vi "Ctrls state & value on Start-Stop.vi"(8 "error in (no error)":errorcluster, 11 "Queue data":T1) -> (0 "error out":errorcluster)   [LabVIEW 2017]
uses:
  Typedefs/Next state queue data.ctl
  Typedefs/Start-Stop Enum.ctl
  Typedefs/Top level VI states.ctl
  Typedefs/Read Write Enum.ctl
  Typedefs/Set Main VI cursor.ctl
  Global Variables/gl_UI Ctrl Refs.vi
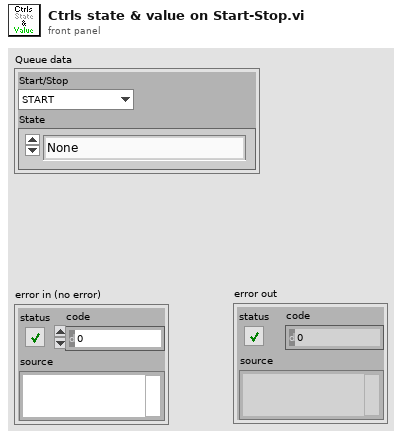
[diagram p1: front panel]
types:
  T1 = typedef "Next state queue data.ctl" = cluster{"Start/Stop":T2, "State":T3}
  T2 = typedef "Start-Stop Enum.ctl" = enum16{"START", "STOP"}
  T3 = typedef "Top level VI states.ctl" = enum16{"None", "Initialise UI", "<STACK PROTOCOL STATES>", "AOL Zstack-START", "AOL Zstack-STOP", "Motor Zstack-START", "Motor Zstack-STOP", "<ACQUISITION PROTOCOL STATES> ", "Functional Acquisition-START", "Functional Acquisition-STOP", "Single Plane Acquisition-START", "Single Plane Acquisition-STOP", "Volume Acquisition-START", "Volume Acquisition-STOP", "<LIVE IMAGING PROTOCOL STATES>", "Live Imaging-START", "Live Imaging-STOP", "Live Plane Imaging-START", "Live Plane Imaging-STOP", "Live Volume Imaging-START", "Live Volume Imaging-STOP", "<MOVEMENT CORRECTION PROTOCOL STATES>", "EXIT"}
  T4 = enum8{"Enabled", "Disabled", "Disabled and Grayed Out"}
  T5 = typedef "Read Write Enum.ctl" = enum16{"Read", "Write"}
  T6 = typedef "UI ctrl refs cluster.ctl" = cluster{"Top level VI path":path, "Top level VI ref":refnum<vi>, "User menu ref":refnum<k9>, "Sub Panel control":refnum<vi>, "Imaging Param Tab":refnum<vi>, "Occurrence-Start drivers":refnum<k4>, "Occurrence-Speed logging initialised":refnum<k4>, "Occurrence-XYZ stage initialised":refnum<k4>, "Exit button":refnum<vi>, "Status ind":refnum<vi>, "Set as origin":refnum<vi>, "Speed Logging":refnum<vi>, "Time Lapse":refnum<vi>, "Live Imaging":refnum<vi>, "AOL Z Stack":refnum<vi>, "Motor Z Stack":refnum<vi>, "Funct Acq button":refnum<vi>, "Hard Shutter":refnum<vi>, "Virtual Shutter":refnum<vi>, "Laser Power":refnum<vi>, "AOL Mode":refnum<vi>, "Frame Size":refnum<vi>, "Field of View":refnum<vi>, "Dwell Time":refnum<vi>, "Zoom":refnum<vi>, "AOL Z":refnum<vi>, "Objective":refnum<vi>, "Axis":refnum<vi>, "Paths & Names":refnum<vi>, "Experiment folder path (ind.)":refnum<vi>, "Last State (Ind.)":refnum<vi>, "Averages":refnum<vi>, "Angle (degrees)":refnum<vi>, "X centre":refnum<vi>, "Y centre":refnum<vi>, "Plane Mode":refnum<vi>, "# Planes":refnum<vi>, "Z Start":refnum<vi>, "Z Stop":refnum<vi>, "Z Step":refnum<vi>, "PMT 1":refnum<vi>, "PMT 2":refnum<vi>, "Stage XYZ Position":refnum<vi>, "Pockels@Z Start":refnum<vi>, "Pockels@Z Stop":refnum<vi>, "Obtain Z Start":refnum<vi>, "Obtain Z Stop":refnum<vi>, "Live stim.trig.period":refnum<vi>, "Live stim.trig.enable":refnum<vi>, "XY Stage Move":refnum<vi>, "Funct. Acq. Pockels Modulation":refnum<vi>, "Enable Video Recording":refnum<vi>, "Video Record-Live Imaging":refnum<vi>, "Video Record-Funct acq":refnum<vi>, "AOL Z-stack Chirps Ready (ind)":refnum<vi>, "Target time between mov.cor. ref triggers (ms)":refnum<vi>, "Funct. Acq. Ref frame save":refnum<vi>, "Show ref plots window":refnum<vi>, "Center freq ind (nm)":refnum<vi>, "Pickup mode (ind)":refnum<vi>, "Logging queue (ind)":refnum<vi>, "Back aperture power (ind.)":refnum<vi>, "Power after objective (ind.)":refnum<vi>, "Switch user":refnum<vi>, "Ls1 Conn. Status":refnum<vi>, "Ls1Tuning Status":refnum<vi>, "Ls1 Faults":refnum<vi>, "Ls1 Connection":refnum<vi>, "Ls1 Mode":refnum<vi>, "Ls1 POWER [mW]":refnum<vi>, "Ls1Shutter":refnum<vi>, "Ls1 Wavelength":refnum<vi>, "Ls1 Note":refnum<vi>, "Ls1 Confirm Wav":refnum<vi>, "Ls1 PreChrp Prism1":refnum<vi>, "Ls1 PreChrp Prism2":refnum<vi>, "Ls1 wav top Ind":refnum<vi>, "Ls1 power top Ind":refnum<vi>, "Ls1 Pump peak Hold":refnum<vi>, "Ls1 Status Ind":refnum<vi>, "Ls1 wav cancel":refnum<vi>, "Experiment Type":refnum<vi>, "Biology Information":refnum<vi>}
  T7 = typedef "Set Main VI cursor.ctl" = enum16{"Release busy cursor", "Set busy cursor"}
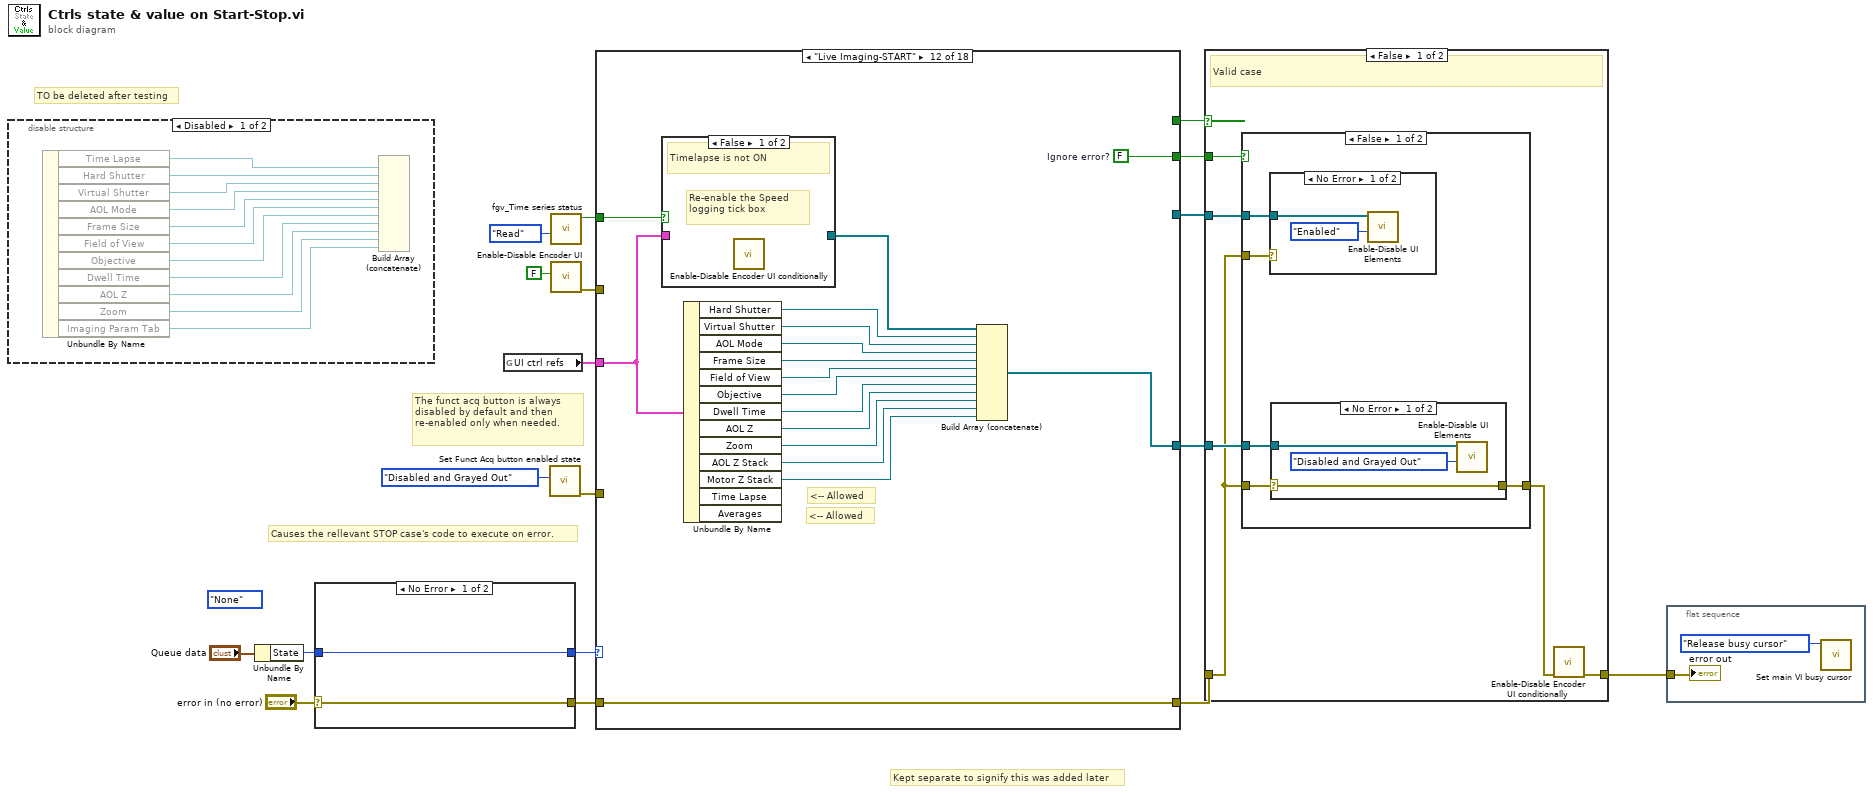
[diagram p0: block diagram]
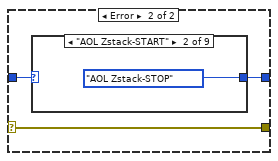
[diagram p3: hidden frame]
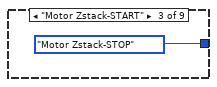
[diagram p5: hidden frame]
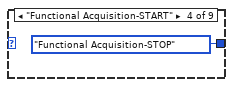
[diagram p6: hidden frame]
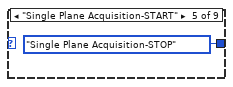
[diagram p7: hidden frame]
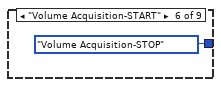
[diagram p8: hidden frame]
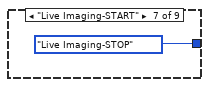
[diagram p9: hidden frame]
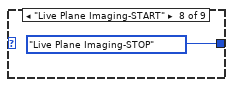
[diagram p10: hidden frame]
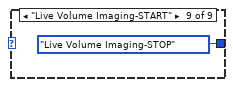
[diagram p11: hidden frame]
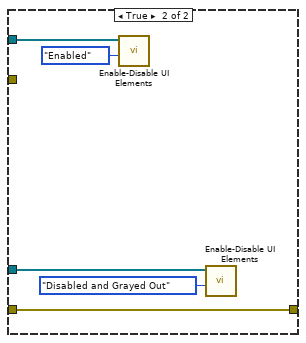
[diagram p14: hidden frame]
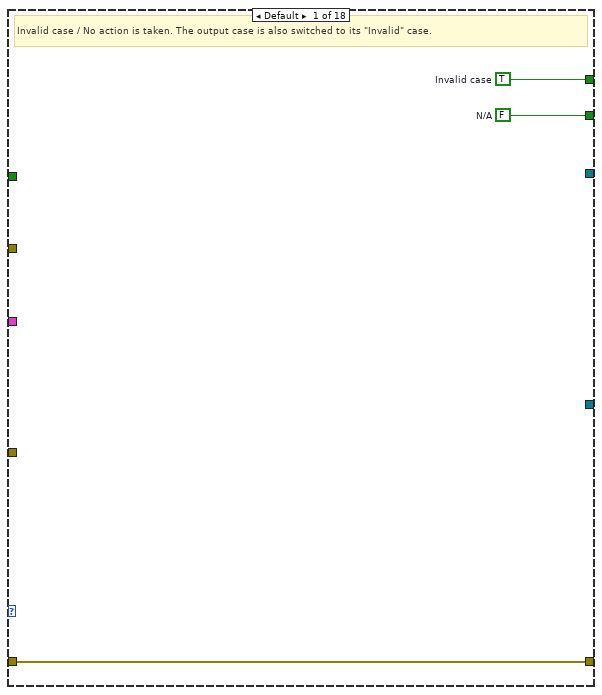
[diagram p16: hidden frame]
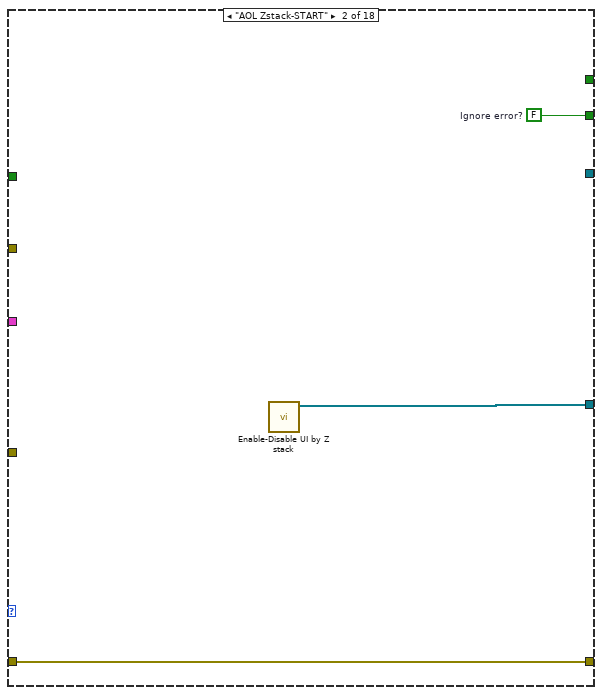
[diagram p17: hidden frame]
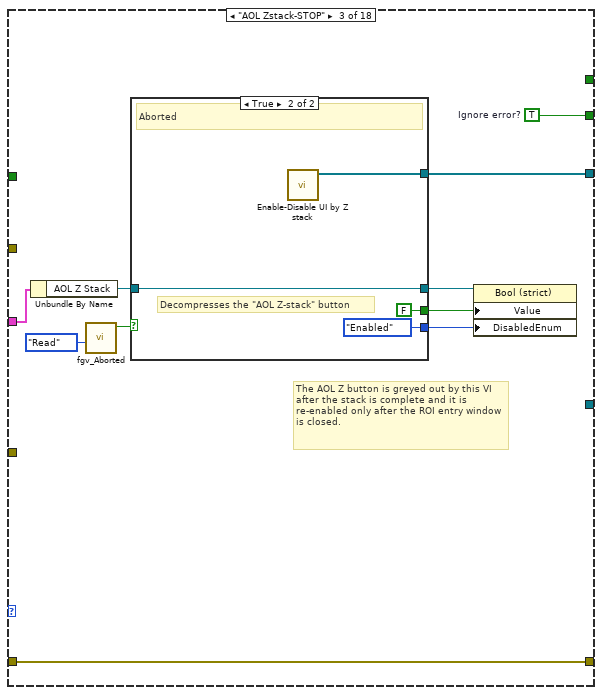
[diagram p18: hidden frame]
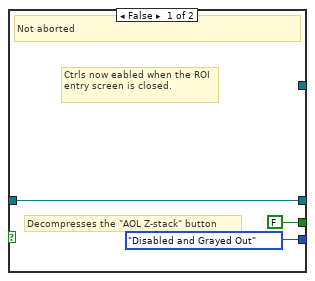
[diagram p19: hidden frame]
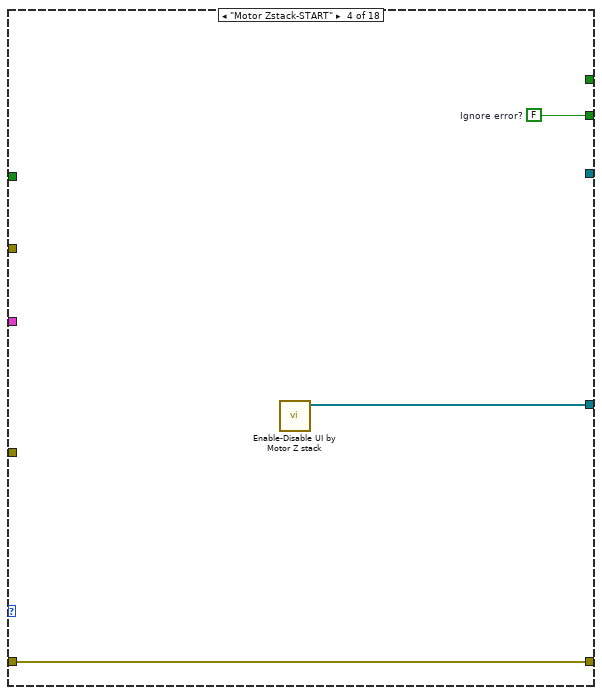
[diagram p20: hidden frame]
diagram:
  (unwired) Top_level_VI_states."None" ("State")
  # "TO be deleted after testing"
  # "Kept separate to signify this was added later"
  # "The funct acq button is always disabled by default and then re-enabled only when needed."
  # "Causes the rellevant STOP case's code to execute on error."
  n1 = disable-structure shown="Disabled" {
    frame Disabled {
      n2 = Unbundle By Name() -> ("Time Lapse"=w20:refnum<vi>, "Hard Shutter"=w22:refnum<vi>, "Virtual Shutter"=w23:refnum<vi>, "AOL Mode"=w24:refnum<vi>, "Frame Size"=w25:refnum<vi>, "Field of View"=w26:refnum<vi>, "Objective"=w27:refnum<vi>, "Dwell Time"=w28:refnum<vi>, "AOL Z"=w29:refnum<vi>, "Zoom"=w30:refnum<vi>, "Imaging Param Tab"=w21:refnum<vi>)  [unwired: 1 in]
      n3 = Build Array (concatenate)(w20, w22, w23, w24, w25, w26, w27, w28, w29, w30, w21) -> (w19:refnum<vi>[])  [unwired: 1 out]
    }
    frame Enabled {
    }
  }
  n4 = Unbundle By Name("Queue data") -> ("State"=w10:T3)
  n5 = case shown="No Error" "error in (no error)" {
    selector: "error in (no error)" -> [w31 w35]
    tunnel: w10 -> [w32 w34]
    tunnel: [w32 w33] -> w8
    tunnel: [w31 w35] -> w4
    frame No Error {
    }
    frame Error {
      n6 = case shown="\"AOL Zstack-START\"" w34 {
        selector: w34 -> [w36 _ _ _ _ _ _ _ _]
        tunnel: [w36 Top_level_VI_states."AOL Zstack-STOP" ("State") Top_level_VI_states."Motor Zstack-STOP" ("State") Top_level_VI_states."Functional Acquisition-STOP" ("State") Top_level_VI_states."Single Plane Acquisition-STOP" ("State") Top_level_VI_states."Volume Acquisition-STOP" ("State") Top_level_VI_states."Live Imaging-STOP" ("State") Top_level_VI_states."Live Plane Imaging-STOP" ("State") Top_level_VI_states."Live Volume Imaging-STOP" ("State")] -> w33
        frame Default {
        }
        frame "AOL Zstack-START" {
        }
        frame "Motor Zstack-START" {
        }
        frame "Functional Acquisition-START" {
        }
        frame "Single Plane Acquisition-START" {
        }
        frame "Volume Acquisition-START" {
        }
        frame "Live Imaging-START" {
        }
        frame "Live Plane Imaging-START" {
        }
        frame "Live Volume Imaging-START" {
        }
      }
    }
  }
  n7 = global read "gl_UI Ctrl Refs.vi" "UI ctrl refs"() -> (w18:T6)
  n8 = call "Set Funct Acq button enabled state.vi"("Disabled"=T4."Disabled and Grayed Out") -> ("error out"=w6:errorcluster)  [unwired: 10 in]
  n9 = call "fgv_Time series status.vi"("Function"=Read_Write_Enum."Read") -> ("Timelapse?"=w11:bool)  [unwired: 10 in]
  n10 = call "Enable-Disable Encoder UI.vi"("Cam VidRec.VidRec available"=FALSE) -> ("error out"=w1:errorcluster)  [unwired: 10 in]
  n11 = case "Message Cases" shown="\"Live Imaging-START\"" w8 {
    tunnel: w18 -> [_ _ w53 _ w72 w91 w112 w132 w151 w170 w188 w205 w224 w242 w259 w273 w291 w306]
    tunnel: [_ _ w56 _ w71 _ w122 _ w160 _ w186 _ w232 _ w263 _ w294 _] -> w17
    tunnel: [w47 _ _ _ _ _ _ _ _ _ _ _ _ _ _ _ _ _] -> w15
    tunnel: [_ w49 _ w70 _ w93 _ w141 _ w176 _ w213 _ w247 _ w278 _ w308] -> w14
    tunnel: [w46 w50 w60 w69 w80 w92 w121 w140 w159 w175 w204 w212 w231 w246 w262 w277 w293 w307] -> w13
    tunnel: w11 -> [_ _ _ _ _ _ _ _ _ _ _ w208 _ w245 _ w276 _ w305]
    tunnel: w6 -> [_ _ _ _ _ _ _ _ _ _ _ _ _ _ _ _ _ _]
    tunnel: w4 -> [w45 w48 w59 w68 w79 w88 w113 w133 w152 w171 w203 w206 w225 w243 w260 w274 w292 w304]
    tunnel: [w45 w48 w59 w68 w79 w88 w113 w133 w152 w171 w203 w206 w225 w243 w260 w274 w292 w304] -> w3
    tunnel: w1 -> [_ _ _ _ _ _ _ _ _ _ _ _ _ _ _ _ _ _]
    frame Default {
      w46 = FALSE  # N/A
      w47 = TRUE  # Invalid case
      # "Invalid case / No action is taken. The output case is also switched to its \"Invalid\" case."
    }
    frame "AOL Zstack-START" {
      w50 = FALSE  # Ignore error?
      n12 = call "Enable-Disable UI by Z stack.vi"() -> ("Controls refs to enable/disable"=w49:refnum<vi>[])  [unwired: 11 in]
    }
    frame "AOL Zstack-STOP" {
      w60 = TRUE  # Ignore error?
      # "The AOL Z button is greyed out by this VI after the stack is complete and it is re-enabled only after the ROI entry window is closed."
      n13 = Unbundle By Name(w53) -> ("AOL Z Stack"=w52:refnum<vi>)
      n14 = call "fgv_Aborted.vi"("Function"=Read_Write_Enum."Read") -> ("Funct Acq Aborted?"=w57:bool)  [unwired: 9 in, 1 out]
      n15 = case shown="True" w57 {
        tunnel: [_ w67] -> w56
        tunnel: [FALSE ("Value") FALSE ("Value")] -> w55
        tunnel: [T4."Disabled and Grayed Out" ("Disabled") T4."Enabled" ("Disabled")] -> w54
        tunnel: w52 -> [w62 w66]
        tunnel: [w62 w66] -> w51
        frame False {
          # "Ctrls now eabled when the ROI entry screen is closed."
          # "Decompresses the \"AOL Z-stack\" button"
          # "Not aborted"
        }
        frame True {
          # "Decompresses the \"AOL Z-stack\" button"
          # "Aborted"
          n16 = call "Enable-Disable UI by Z stack.vi"() -> ("Controls refs to enable/disable"=w67:refnum<vi>[])  [unwired: 11 in]
        }
      }
      n17 = property class="Bool (strict)"(reference=w51, "Value"=w55, "DisabledEnum"=w54) -> ()  [unwired: 1 in, 2 out]
    }
    frame "Motor Zstack-START" {
      w69 = FALSE  # Ignore error?
      n18 = call "Enable-Disable UI by Motor Z stack.vi"() -> ("Controls to disable"=w70:refnum<vi>[])  [unwired: 11 in]
    }
    frame "Motor Zstack-STOP" {
      w80 = TRUE  # Ignore error?
      # "The Motor Z button is greyed out by this VI after the stack is complete and it is re-enabled only after the ROI entry window is closed."
      n19 = Unbundle By Name(w72) -> ("Motor Z Stack"=w77:refnum<vi>)
      n20 = call "fgv_Aborted.vi"("Function"=Read_Write_Enum."Read") -> ("Funct Acq Aborted?"=w74:bool)  [unwired: 9 in, 1 out]
      n21 = case shown="False" w74 {
        tunnel: [_ w84] -> w71
        tunnel: [FALSE ("Value") FALSE ("Value")] -> w75
        tunnel: [T4."Disabled and Grayed Out" ("Disabled") T4."Enabled" ("Disabled")] -> w76
        tunnel: w77 -> [w82 w87]
        tunnel: [w82 w87] -> w78
        frame False {
          # "Ctrls now eabled when the ROI entry screen is closed."
          # "Decompresses the \"AOL Z-stack\" button"
          # "Not aborted"
        }
        frame True {
          # "Decompresses the \"Motor Z-stack\" button"
          # "Aborted"
          n22 = call "Enable-Disable UI by Motor Z stack.vi"() -> ("Controls to disable"=w84:refnum<vi>[])  [unwired: 11 in]
        }
      }
      n23 = property class="Bool (strict)"(reference=w78, "Value"=w75, "DisabledEnum"=w76) -> ()  [unwired: 1 in, 2 out]
    }
    frame "Functional Acquisition-START" {
      w92 = FALSE  # Ignore error?
      # "The funct acq button's state is explicitly set by this VI, throughout the software."
      n24 = call "Set Funct Acq button enabled state.vi"("Disabled"=T4."Enabled") -> ("error out"=w89:errorcluster)  [unwired: 10 in]
      n25 = flat-sequence {
        tunnel: [w110] -> w93
        tunnel: w91 -> [w94]
        tunnel: w89 -> [_]
        frame #0 {
          n26 = Unbundle By Name(w94) -> ("Time Lapse"=w99:refnum<vi>, "Imaging Param Tab"=w100:refnum<vi>, "Hard Shutter"=w101:refnum<vi>, "Virtual Shutter"=w102:refnum<vi>, "AOL Mode"=w103:refnum<vi>, "Frame Size"=w104:refnum<vi>, "Field of View"=w105:refnum<vi>, "Objective"=w106:refnum<vi>, "Dwell Time"=w107:refnum<vi>, "AOL Z"=w108:refnum<vi>, "Zoom"=w109:refnum<vi>, "Live Imaging"=w97:refnum<vi>, "AOL Z Stack"=w96:refnum<vi>, "Motor Z Stack"=w95:refnum<vi>)
          n27 = call "Time series conditional disable ctrl refs.vi"("UI ctrl refs"=w94) -> ("Ctrl refs"=w98:refnum<vi>[])  [unwired: 10 in]
          n28 = Build Array (concatenate)(w98, w99, w100, w101, w102, w103, w104, w105, w106, w107, w108, w109, w97, w96, w95) -> (w110:refnum<vi>[])
        }
      }
    }
    frame "Functional Acquisition-STOP" {
      w121 = TRUE  # Ignore error?
      # "Decompresses the \"funct. acq.\" button"
      # "Controls enabled when Live Imaging is stopped"
      n29 = Unbundle By Name(w112) -> ("Time Lapse"=w119:refnum<vi>, "Hard Shutter"=w123:refnum<vi>, "Virtual Shutter"=w124:refnum<vi>, "AOL Mode"=w125:refnum<vi>, "Frame Size"=w126:refnum<vi>, "Field of View"=w127:refnum<vi>, "Objective"=w128:refnum<vi>, "Dwell Time"=w129:refnum<vi>, "AOL Z"=w130:refnum<vi>, "Zoom"=w131:refnum<vi>, "Imaging Param Tab"=w120:refnum<vi>, "Live Imaging"=w118:refnum<vi>, "AOL Z Stack"=w117:refnum<vi>, "Motor Z Stack"=w116:refnum<vi>)
      n30 = call "Time series conditional disable ctrl refs.vi"("UI ctrl refs"=w112) -> ("Ctrl refs"=w111:refnum<vi>[])  [unwired: 10 in]
      n31 = call "Set Funct Acq button value.vi"("Functional Acquisition button's new value"=FALSE ("Value")) -> ()  [unwired: 10 in, 1 out]
      n32 = call "Set Funct Acq button enabled state.vi"("Disabled"=T4."Enabled") -> ()  [unwired: 10 in, 1 out]
      n33 = Build Array (concatenate)(w119, w123, w124, w125, w126, w127, w128, w129, w130, w131, w120, w118, w117, w116, w111) -> (w122:refnum<vi>[])
    }
    frame "Single Plane Acquisition-START" {
      w140 = FALSE  # Ignore error?
      # "Not in use - placeholder only"
      n34 = Unbundle By Name(w132) -> ("Time Lapse"=w138:refnum<vi>, "Imaging Param Tab"=w139:refnum<vi>, "Hard Shutter"=w142:refnum<vi>, "Virtual Shutter"=w143:refnum<vi>, "AOL Mode"=w144:refnum<vi>, "Frame Size"=w145:refnum<vi>, "Field of View"=w146:refnum<vi>, "Objective"=w147:refnum<vi>, "Dwell Time"=w148:refnum<vi>, "AOL Z"=w149:refnum<vi>, "Zoom"=w150:refnum<vi>, "AOL Z Stack"=w136:refnum<vi>, "Motor Z Stack"=w135:refnum<vi>, "Live Imaging"=w134:refnum<vi>)
      n35 = call "Time series conditional disable ctrl refs.vi"("UI ctrl refs"=w132) -> ("Ctrl refs"=w137:refnum<vi>[])  [unwired: 10 in]
      n36 = Build Array (concatenate)(w137, w138, w139, w142, w143, w144, w145, w146, w147, w148, w149, w150, w136, w135, w134) -> (w141:refnum<vi>[])
    }
    frame "Single Plane Acquisition-STOP" {
      w159 = TRUE  # Ignore error?
      # "Not in use place holder only"
      n37 = Unbundle By Name(w151) -> ("Time Lapse"=w157:refnum<vi>, "Hard Shutter"=w161:refnum<vi>, "Virtual Shutter"=w162:refnum<vi>, "AOL Mode"=w163:refnum<vi>, "Frame Size"=w164:refnum<vi>, "Field of View"=w165:refnum<vi>, "Objective"=w166:refnum<vi>, "Dwell Time"=w167:refnum<vi>, "AOL Z"=w168:refnum<vi>, "Zoom"=w169:refnum<vi>, "Imaging Param Tab"=w158:refnum<vi>, "AOL Z Stack"=w156:refnum<vi>, "Motor Z Stack"=w155:refnum<vi>, "Live Imaging"=w154:refnum<vi>)
      n38 = call "Time series conditional disable ctrl refs.vi"("UI ctrl refs"=w151) -> ("Ctrl refs"=w153:refnum<vi>[])  [unwired: 10 in]
      n39 = Build Array (concatenate)(w153, w157, w161, w162, w163, w164, w165, w166, w167, w168, w169, w158, w156, w155, w154) -> (w160:refnum<vi>[])
    }
    frame "Volume Acquisition-START" {
      w175 = FALSE  # Ignore error?
      # "Not in use place holder only"
      n40 = Unbundle By Name(w170) -> ("Time Lapse"=w173:refnum<vi>, "Imaging Param Tab"=w174:refnum<vi>, "Hard Shutter"=w177:refnum<vi>, "Virtual Shutter"=w178:refnum<vi>, "AOL Mode"=w179:refnum<vi>, "Frame Size"=w180:refnum<vi>, "Field of View"=w181:refnum<vi>, "Objective"=w182:refnum<vi>, "Dwell Time"=w183:refnum<vi>, "AOL Z"=w184:refnum<vi>, "Zoom"=w185:refnum<vi>)
      n41 = call "Time series conditional disable ctrl refs.vi"("UI ctrl refs"=w170) -> ("Ctrl refs"=w172:refnum<vi>[])  [unwired: 10 in]
      n42 = Build Array (concatenate)(w172, w173, w174, w177, w178, w179, w180, w181, w182, w183, w184, w185) -> (w176:refnum<vi>[])
    }
    frame "Volume Acquisition-STOP" {
      w204 = TRUE  # Ignore error?
      # "Not in use place holder only"
      n43 = call "Time series conditional disable ctrl refs.vi"("UI ctrl refs"=w188) -> ("Ctrl refs"=w187:refnum<vi>[])  [unwired: 10 in]
      n44 = Unbundle By Name(w188) -> ("Time Lapse"=w192:refnum<vi>, "Hard Shutter"=w194:refnum<vi>, "Virtual Shutter"=w195:refnum<vi>, "AOL Mode"=w196:refnum<vi>, "Frame Size"=w197:refnum<vi>, "Field of View"=w198:refnum<vi>, "Objective"=w199:refnum<vi>, "Dwell Time"=w200:refnum<vi>, "AOL Z"=w201:refnum<vi>, "Zoom"=w202:refnum<vi>, "Imaging Param Tab"=w193:refnum<vi>, "Live Imaging"=w191:refnum<vi>, "AOL Z Stack"=w190:refnum<vi>, "Motor Z Stack"=w189:refnum<vi>)
      n45 = Build Array (concatenate)(w187, w192, w194, w195, w196, w197, w198, w199, w200, w201, w202, w193, w191, w190, w189) -> (w186:refnum<vi>[])
    }
    frame "Live Imaging-START" {
      w212 = FALSE  # Ignore error?
      # "<-- Allowed"
      # "<-- Allowed"
      n46 = case shown="False" w208 {
        tunnel: w205 -> [_ w223]
        tunnel: [_ w222] -> w209
        frame False {
          # "Re-enable the Speed logging tick box"
          # "Timelapse is not ON"
          n47 = call "Enable-Disable Encoder UI conditionally.vi"() -> ()  [unwired: 11 in, 1 out]
        }
        frame True {
          # "Time-lapse is ON"
          n48 = call "Time series conditional disable ctrl refs.vi"("UI ctrl refs"=w223) -> ("Ctrl refs"=w222:refnum<vi>[])  [unwired: 10 in]
        }
      }
      n49 = Unbundle By Name(w205) -> ("Hard Shutter"=w207:refnum<vi>, "Virtual Shutter"=w214:refnum<vi>, "AOL Mode"=w215:refnum<vi>, "Frame Size"=w216:refnum<vi>, "Field of View"=w217:refnum<vi>, "Objective"=w218:refnum<vi>, "Dwell Time"=w219:refnum<vi>, "AOL Z"=w220:refnum<vi>, "Zoom"=w221:refnum<vi>, "AOL Z Stack"=w211:refnum<vi>, "Motor Z Stack"=w210:refnum<vi>)  [unwired: 2 out]
      n50 = Build Array (concatenate)(w209, w207, w214, w215, w216, w217, w218, w219, w220, w221, w211, w210) -> (w213:refnum<vi>[])
    }
    frame "Live Imaging-STOP" {
      w231 = TRUE  # Ignore error?
      # "<-- Allowed"
      # "Decompresses the \"Live Imaging.\" button"
      # "<-- Allowed"
      n51 = Unbundle By Name(w224) -> ("Live Imaging"=w228:refnum<vi>)
      n52 = Unbundle By Name(w224) -> ("Hard Shutter"=w233:refnum<vi>, "Virtual Shutter"=w234:refnum<vi>, "AOL Mode"=w235:refnum<vi>, "Frame Size"=w236:refnum<vi>, "Field of View"=w237:refnum<vi>, "Objective"=w238:refnum<vi>, "Dwell Time"=w239:refnum<vi>, "AOL Z"=w240:refnum<vi>, "Zoom"=w241:refnum<vi>, "AOL Z Stack"=w230:refnum<vi>, "Motor Z Stack"=w229:refnum<vi>)  [unwired: 2 out]
      n53 = call "Time series conditional disable ctrl refs.vi"("UI ctrl refs"=w224) -> ("Ctrl refs"=w226:refnum<vi>[])  [unwired: 10 in]
      n54 = property class="Bool (strict)"(reference=w228, "Value"=FALSE) -> ()  [unwired: 1 in, 2 out]
      n55 = Build Array (concatenate)(w226, w233, w234, w235, w236, w237, w238, w239, w240, w241, w230, w229) -> (w232:refnum<vi>[])
    }
    frame "Live Plane Imaging-START" {
      w246 = FALSE  # Ignore error?
      # "Not in use place holder only"
      n56 = case shown="True" w245 {
        tunnel: w242 -> [_ w258]
        tunnel: [_ w257] -> w244
        frame False {
          # "Re-enable the Speed logging tick box"
          # "Timelapse is not ON"
          n57 = call "Enable-Disable Encoder UI conditionally.vi"() -> ()  [unwired: 11 in, 1 out]
        }
        frame True {
          # "Time-lapse is ON"
          n58 = call "Time series conditional disable ctrl refs.vi"("UI ctrl refs"=w258) -> ("Ctrl refs"=w257:refnum<vi>[])  [unwired: 10 in]
        }
      }
      n59 = Unbundle By Name(w242) -> ("Hard Shutter"=w248:refnum<vi>, "Virtual Shutter"=w249:refnum<vi>, "AOL Mode"=w250:refnum<vi>, "Frame Size"=w251:refnum<vi>, "Field of View"=w252:refnum<vi>, "Objective"=w253:refnum<vi>, "Dwell Time"=w254:refnum<vi>, "AOL Z"=w255:refnum<vi>, "Zoom"=w256:refnum<vi>)
      n60 = Build Array (concatenate)(w244, w248, w249, w250, w251, w252, w253, w254, w255, w256) -> (w247:refnum<vi>[])
    }
    frame "Live Plane Imaging-STOP" {
      w262 = TRUE  # Ignore error?
      # "Not in use place holder only"
      n61 = Unbundle By Name(w259) -> ("Hard Shutter"=w264:refnum<vi>, "Virtual Shutter"=w265:refnum<vi>, "AOL Mode"=w266:refnum<vi>, "Frame Size"=w267:refnum<vi>, "Field of View"=w268:refnum<vi>, "Objective"=w269:refnum<vi>, "Dwell Time"=w270:refnum<vi>, "AOL Z"=w271:refnum<vi>, "Zoom"=w272:refnum<vi>)
      n62 = call "Time series conditional disable ctrl refs.vi"("UI ctrl refs"=w259) -> ("Ctrl refs"=w261:refnum<vi>[])  [unwired: 10 in]
      n63 = Build Array (concatenate)(w261, w264, w265, w266, w267, w268, w269, w270, w271, w272) -> (w263:refnum<vi>[])
    }
    frame "Live Volume Imaging-START" {
      w277 = FALSE  # Ignore error?
      # "Not in use place holder only"
      n64 = Unbundle By Name(w273) -> ("Hard Shutter"=w279:refnum<vi>, "Virtual Shutter"=w280:refnum<vi>, "AOL Mode"=w281:refnum<vi>, "Frame Size"=w282:refnum<vi>, "Field of View"=w283:refnum<vi>, "Objective"=w284:refnum<vi>, "Dwell Time"=w285:refnum<vi>, "AOL Z"=w286:refnum<vi>, "Zoom"=w287:refnum<vi>)
      n65 = case shown="False" w276 {
        tunnel: w273 -> [_ w289]
        tunnel: [_ w288] -> w275
        frame False {
          # "Re-enable the Speed logging tick box"
          # "Time-lapse is not ON"
          n66 = call "Enable-Disable Encoder UI conditionally.vi"() -> ()  [unwired: 11 in, 1 out]
        }
        frame True {
          # "Time-lapse is ON"
          n67 = call "Time series conditional disable ctrl refs.vi"("UI ctrl refs"=w289) -> ("Ctrl refs"=w288:refnum<vi>[])  [unwired: 10 in]
        }
      }
      n68 = Build Array (concatenate)(w275, w279, w280, w281, w282, w283, w284, w285, w286, w287) -> (w278:refnum<vi>[])
    }
    frame "Live Volume Imaging-STOP" {
      w293 = TRUE  # Ignore error?
      # "Not in use place holder only"
      n69 = Unbundle By Name(w291) -> ("Hard Shutter"=w295:refnum<vi>, "Virtual Shutter"=w296:refnum<vi>, "AOL Mode"=w297:refnum<vi>, "Frame Size"=w298:refnum<vi>, "Field of View"=w299:refnum<vi>, "Objective"=w300:refnum<vi>, "Dwell Time"=w301:refnum<vi>, "AOL Z"=w302:refnum<vi>, "Zoom"=w303:refnum<vi>)
      n70 = call "Time series conditional disable ctrl refs.vi"("UI ctrl refs"=w291) -> ("Ctrl refs"=w290:refnum<vi>[])  [unwired: 10 in]
      n71 = Build Array (concatenate)(w295, w296, w297, w298, w299, w300, w301, w302, w303, w290) -> (w294:refnum<vi>[])
    }
    frame "EXIT" {
      w307 = FALSE  # Ignore error?
      n72 = disable-structure shown="Disabled" {
        disable-tunnel: [w315 _] -> w308
        disable-tunnel: w306 -> [w312 _]
        disable-tunnel: w305 -> [w310 _]
        frame Disabled {
          # "<-- Allowed"
          # "<-- Allowed"
          # "Controls disabled during Live Imaging"
          n73 = case shown="False" w310 {
            tunnel: w312 -> [_ w325]
            tunnel: [_ w324] -> w311
            frame False {
              # "Re-enable the Speed logging tick box"
              # "Time-lapse is not ON"
              n74 = call "Enable-Disable Encoder UI conditionally.vi"() -> ()  [unwired: 11 in, 1 out]
            }
            frame True {
              # "Time-lapse is ON"
              n75 = call "Time series conditional disable ctrl refs.vi"("UI ctrl refs"=w325) -> ("Ctrl refs"=w324:refnum<vi>[])  [unwired: 10 in]
            }
          }
          n76 = Unbundle By Name(w312) -> ("Hard Shutter"=w309:refnum<vi>, "Virtual Shutter"=w316:refnum<vi>, "AOL Mode"=w317:refnum<vi>, "Frame Size"=w318:refnum<vi>, "Field of View"=w319:refnum<vi>, "Objective"=w320:refnum<vi>, "Dwell Time"=w321:refnum<vi>, "AOL Z"=w322:refnum<vi>, "Zoom"=w323:refnum<vi>, "AOL Z Stack"=w314:refnum<vi>, "Motor Z Stack"=w313:refnum<vi>)  [unwired: 2 out]
          n77 = Build Array (concatenate)(w311, w309, w316, w317, w318, w319, w320, w321, w322, w323, w314, w313) -> (w315:refnum<vi>[])
        }
        frame Enabled {
        }
      }
    }
  }
  n78 = case shown="False" w15 {
    tunnel: w17 -> [w331 _]
    tunnel: w14 -> [w330 _]
    tunnel: w13 -> [w329 _]
    tunnel: w3 -> [w327 w348]
    tunnel: [w328 w348] -> w5
    frame False {
      # "Valid case"
      n79 = case shown="False" w329 {
        tunnel: w327 -> [w336 _]
        tunnel: w331 -> [w335 w347]
        tunnel: w330 -> [w334 w346]
        tunnel: w327 -> [w333 w343]
        tunnel: [w332 w343] -> w326
        frame False {
          n80 = case shown="No Error" w336 {
            tunnel: w335 -> [w342 _]
            frame No Error {
              n81 = call "Enable-Disable UI Elements.vi"("Enable/Disable"=T4."Enabled", "Ctrl ref's"=w342) -> ()  [unwired: 9 in, 1 out]
            }
            frame Error {
            }
          }
          n82 = case shown="No Error" w333 {
            selector: w333 -> [w337 w340]
            tunnel: w334 -> [w339 _]
            tunnel: [w337 w340] -> w332
            frame No Error {
              n83 = call "Enable-Disable UI Elements.vi"("Enable/Disable"=T4."Disabled and Grayed Out", "Ctrl ref's"=w339) -> ()  [unwired: 9 in, 1 out]
            }
            frame Error {
            }
          }
        }
        frame True {
          n84 = call "Enable-Disable UI Elements.vi"("Enable/Disable"=T4."Enabled", "Ctrl ref's"=w347) -> ()  [unwired: 9 in, 1 out]
          n85 = call "Enable-Disable UI Elements.vi"("Enable/Disable"=T4."Disabled and Grayed Out", "Ctrl ref's"=w346) -> ()  [unwired: 9 in, 1 out]
        }
      }
      n86 = call "Enable-Disable Encoder UI conditionally.vi"("error in"=w326) -> ("error out"=w328:errorcluster)  [unwired: 10 in]
    }
    frame True {
      # "Invalid case"
    }
  }
  n87 = flat-sequence {
    tunnel: w5 -> [w349]
    frame #0 {
      n88 = call "Set main VI busy cursor.vi"("Main VI's cursor"=Set_Main_VI_cursor."Release busy cursor") -> ()  [unwired: 10 in, 1 out]
      "error out" <- w349
    }
  }
